vi "CreatedotNETDataTable.vi"(8 "error in (no error)":errorcluster caption="Fehler (Eingang, kein Fehler)", 11 "LoadConfigurationDataBase Eingang":refnum<class "LoadConfigurationDataBase.lvclass"> caption="DNL_LabVIEW Object in") -> (0 "error out":errorcluster caption="Fehler (Ausgang)", 2 "myDataTable":refnum<k24>, 3 "LoadConfigurationDataBase Ausgang":refnum<class "LoadConfigurationDataBase.lvclass"> caption="DNL_LabVIEW Object out")   [LabVIEW 2013, in "LoadConfigurationDataBase.lvclass"]
uses:
  LoadConfigurationDataBase.lvclass
  System.Data
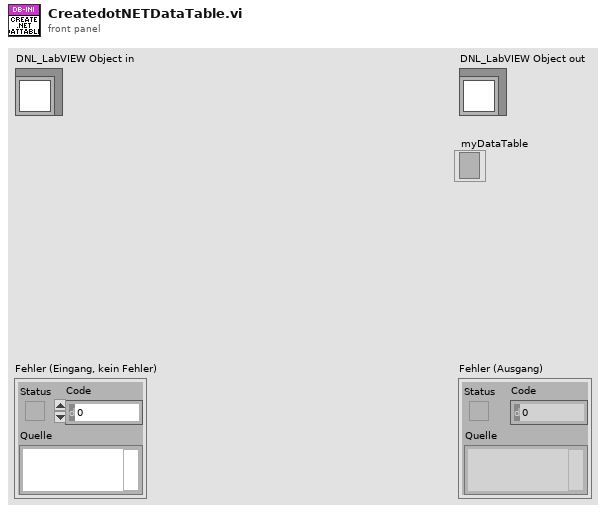
[diagram p1: front panel]
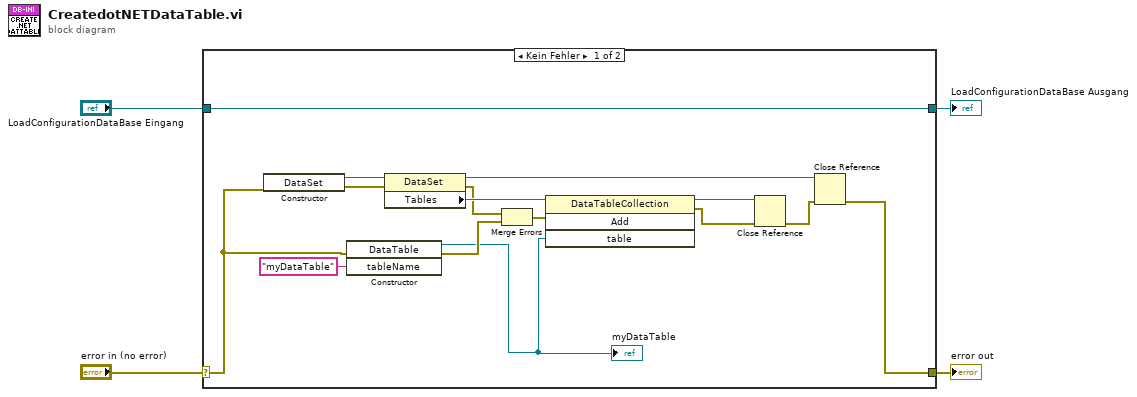
[diagram p0: block diagram]
diagram:
  n1 = case shown="Kein Fehler" "error in (no error)" {
    selector: "error in (no error)" -> [w10 w21]
    tunnel: [w5 w21] -> w3
    tunnel: [w19 w20] -> w1
    tunnel: "LoadConfigurationDataBase Eingang" -> [w19 w20]
    frame No Error {
      n2 = constructor class="DataSet"(error in=w10) -> (reference out=w17:refnum<k24>, error out=w16:errorcluster)  [unwired: 2 in, 1 out]
      n3 = constructor class="DataTable"(error in=w10, "tableName"="myDataTable") -> (reference out=w11:refnum<k24>, error out=w12:errorcluster)  [unwired: 2 in, 2 out]
      "myDataTable" <- w11
      n4 = property class="DataSet"(reference=w17, error in=w16) -> (reference out=w6:refnum<k24>, error out=w14:errorcluster, "Tables"=w15:refnum<k24>)
      n5 = Merge Errors(w14, w12) -> (w13:errorcluster)
      n6 = invoke class="DataTableCollection" method="Add"(reference=w15, error in=w13, "table"=w11) -> (reference out=w9:refnum<k24>, error out=w8:errorcluster)  [unwired: 1 in, 2 out]
      n7 = Close Reference(reference=w9, error in (no error)=w8) -> (error out=w7:errorcluster)
      n8 = Close Reference(reference=w6, error in (no error)=w7) -> (error out=w5:errorcluster)
    }
    frame Error {
    }
  }
  "error out" <- w3
  "LoadConfigurationDataBase Ausgang" <- w1
